vi "debug_temporal_calibration.vi"() -> ()   [LabVIEW 2019]
uses:
  ParametersGlobal.vi
  <vilib>/vision/NI_Vision_Development_Module.lvlib
panel:
  in  "starting frame":i32=43
  out "x-y":i32
  out "Path":path
  out "image #":i32
  out "Camera Input":T1(plugin-control)
  out "32bit integer":i32
  in  "Experiment Folder in":string="C:\\Data\\"
  out "error out":errorcluster
  in  "error in (no error)":errorcluster
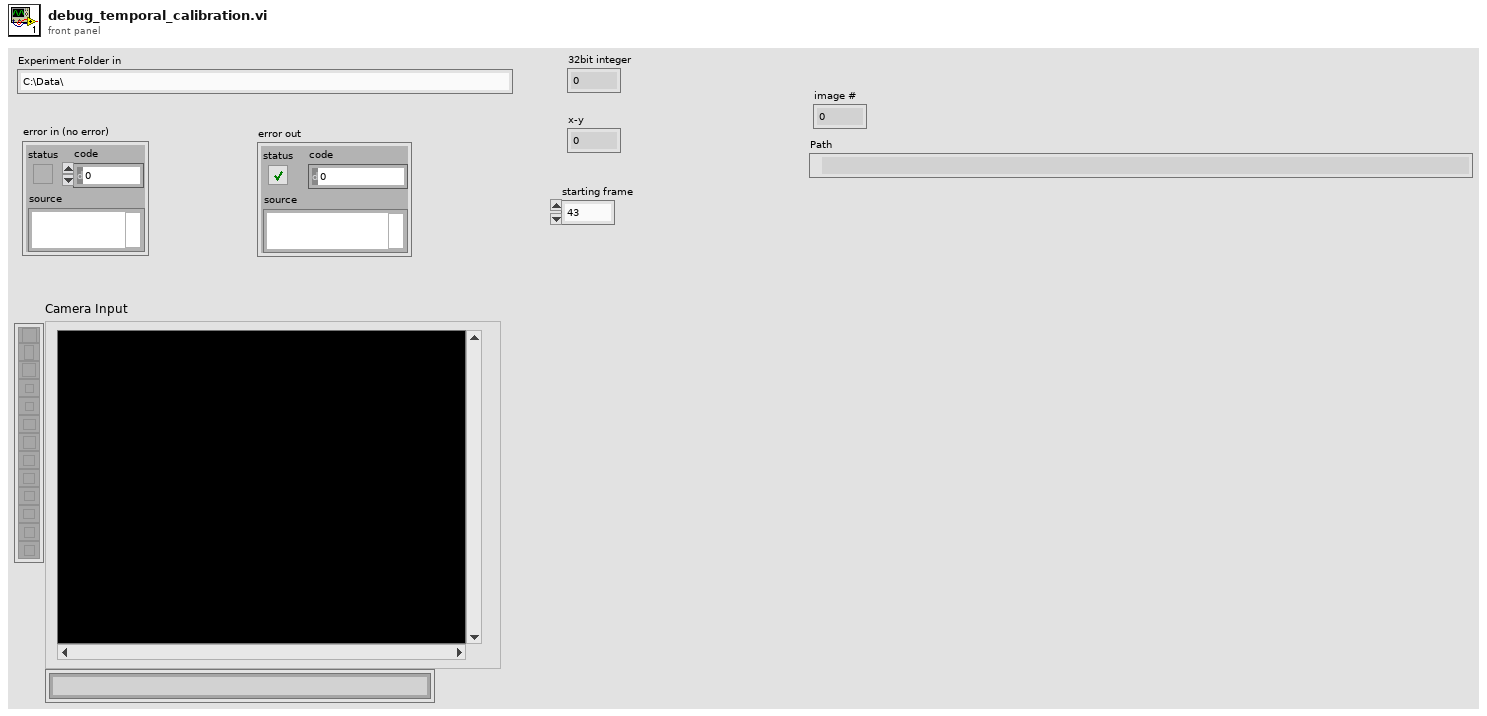
[diagram p1: front panel]
types:
  T1 = typedef "IMAQ Image.ctl" = refnum<image>
  T2 = typedef "Image Type" = u32
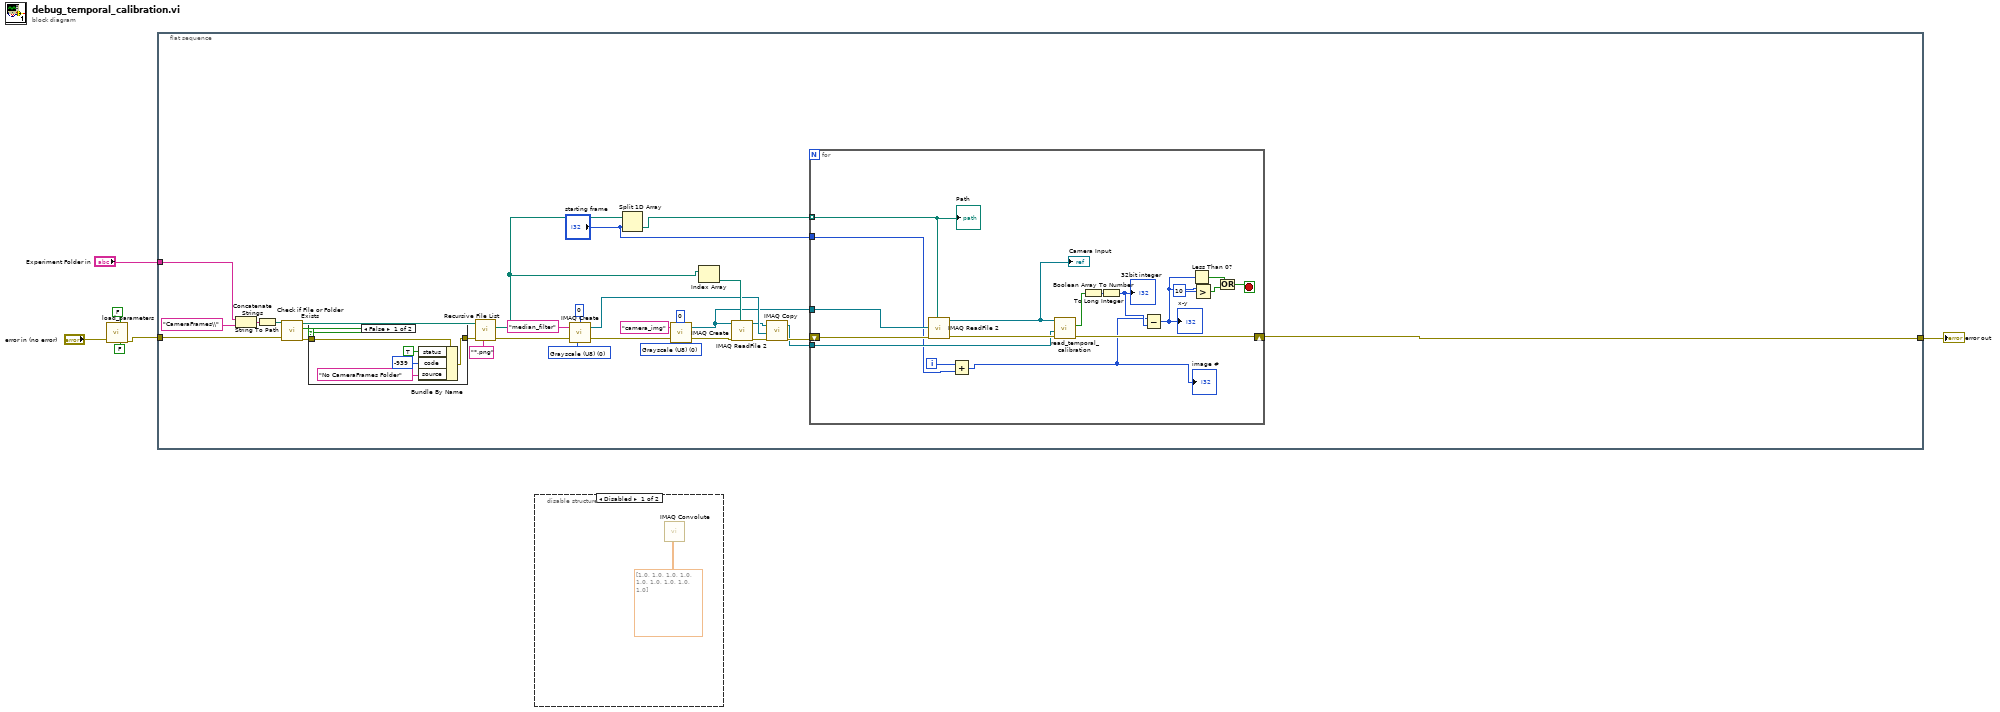
[diagram p0: block diagram]
diagram:
  n1 = call "load_parameters.vi"("Create Data Folder (T)"=FALSE, "Set Up Projector and Camera (T)"=FALSE, "error in (no error)"="error in (no error)") -> ("error out"=w1:errorcluster)  [unwired: 6 in, 2 out]
  n2 = flat-sequence {
    tunnel: [w27] -> w6
    tunnel: "Experiment Folder in" -> [w29]
    tunnel: w1 -> [w19]
    frame #0 {
      w22 = T2 0 items=["Grayscale (U8)", "Grayscale (I16)", "Grayscale (SGL)", "Complex (CSG)", "RGB (U32)", "HSL (U32)", "RGB (U64)", "Grayscale (U16)"] ("Image Type")
      w25 = T2 0 items=["Grayscale (U8)", "Grayscale (I16)", "Grayscale (SGL)", "Complex (CSG)", "RGB (U32)", "HSL (U32)", "RGB (U64)", "Grayscale (U16)"] ("Image Type")
      n3 = Concatenate Strings(w29, "CameraFrames\\" ("string")) -> (w34:string)
      n4 = String To Path(string=w34) -> (path=w33:path)
      n5 = call <vilib>:"Check if File or Folder Exists.vi"("error in (no error)"=w19, "path"=w33) -> ("error out"=w31:errorcluster, "file or folder exists?"=w32:bool, "dup path"=w28:path)  [unwired: 7 in]
      n6 = case shown="False" w32 {
        tunnel: w31 -> [w59 w60]
        tunnel: [w55 w60] -> w30
        frame False {
          n7 = Bundle By Name(cluster=w59, "status"=TRUE, "code"=-939, "source"="No CameraFrames Folder") -> (w55:errorcluster)
        }
        frame True {
        }
      }
      n8 = call <vilib>:"Recursive File List.vi"("pattern"="*.png", "error in (no error)"=w30, "Folder Path"=w28) -> ("error out"=w20:errorcluster, "All Files in Dir"=w9:path[])  [unwired: 4 in, 3 out]
      n9 = call "IMAQ Create"("Border Size"=0, "Image Name"="median_filter", "Image Type"=w22, "error in (no error)"=w20) -> ("New Image"=w13:T1, "error out"=w14:errorcluster)  [unwired: 1 in]
      n10 = Split 1D Array(array=w9, index="starting frame") -> (second subarray=w8:path[])  [unwired: 1 out]
      n11 = call "IMAQ Create"("Border Size"=0, "Image Name"="camera_img", "Image Type"=w25, "error in (no error)"=w14) -> ("New Image"=w11:T1, "error out"=w18:errorcluster)  [unwired: 1 in]
      n12 = Index Array(array=w9) -> (element=w17:path)  [unwired: 1 in]
      n13 = call "IMAQ ReadFile 2"("File Path"=w17, "error in (no error)"=w18, "Image"=w11) -> ("error out"=w16:errorcluster, "Image Out"=w12:T1)  [unwired: 4 in, 3 out]
      n14 = call "IMAQ Copy"("error in (no error)"=w16, "Image Dst"=w13, "Image Src"=w12) -> ("error out"=w15:errorcluster, "Image Dst Out"=w10:T1)  [unwired: 3 in]
      n15 = for {
        tunnel: w8 -> [w54] mode=indexing
        shift-right: [w53] -> w27
        shift-left: w15 -> [w52]
        tunnel: w11 -> [w47]
        tunnel: w10 -> [w46]
        tunnel: "starting frame" -> [w37]
        i -> [w39]
        stop <- w41 stop-if-true
        n16 = call "IMAQ ReadFile 2"("File Path"=w54, "error in (no error)"=w52, "Image"=w47) -> ("error out"=w49:errorcluster, "Image Out"=w48:T1)  [unwired: 4 in, 3 out]
        "Camera Input" <- w48
        n17 = Add(x=w39, y=w37) -> (x+y=w38:i32)
        "image #" <- w38
        n18 = call "read_temporal_calibration.vi"("error in (no error)"=w49, "Median Filtered Image"=w46, "Aquired Image"=w48) -> ("error out"=w53:errorcluster, "Time Bits Decoded"=w51:bool[])  [unwired: 6 in, 1 out]
        n19 = Boolean Array To Number(Boolean array=w51) -> (number=w50:u64)
        n20 = To Long Integer(number=w50) -> (32bit integer=w40:i32)
        "32bit integer" <- w40
        n21 = Subtract(x=w38, y=w40) -> (x-y=w45:i32)
        "x-y" <- w45
        n22 = Less Than 0?(x=w45) -> (x < 0?=w43:bool)
        n23 = Greater?(x=w45, y=10) -> (0:w42:bool)
        n24 = Or(x=w43, y=w42) -> (x .or. y?=w41:bool)
        "Path" <- w54
      }
    }
  }
  n25 = disable-structure shown="Disabled" {
    frame Disabled {
      n26 = call "IMAQ Convolute"("Kernel"=sgl[][] [[1.0, 1.0, 1.0], [1.0, 1.0, 1.0], [1.0, 1.0, 1.0]]) -> ("Image Dst Out"=w61:T1, "error in (no error)"=w63:errorcluster, "Image Src"=w64:T1)  [unwired: 7 in, 1 out]
    }
    frame Enabled {
    }
  }
  "error out" <- w6
